vi "Prepare Config.vi"(8 "Error In":errorcluster, 11 "IConfig In":refnum<class "IConfig.lvclass">) -> (0 "Error Out":errorcluster, 3 "IConfig Out":refnum<class "IConfig.lvclass">)   [LabVIEW 2020, in "IConfig.lvclass"]
uses:
  IConfig.lvclass
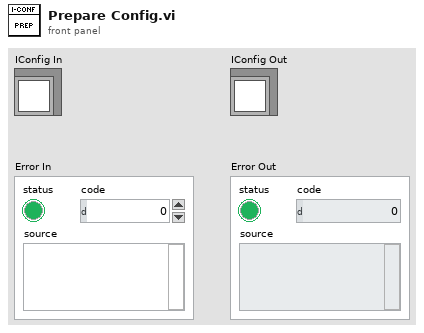
[diagram p1: front panel]
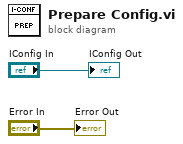
[diagram p0: block diagram]
diagram:
  "Error Out" <- "Error In"
  "IConfig Out" <- "IConfig In"
